vi "XNET String To IO Name (LIN Schedule Entry).vi"(3 "string":string) -> (0 "XNET LIN schedule entry":refnum<k21>)   [LabVIEW 2018]
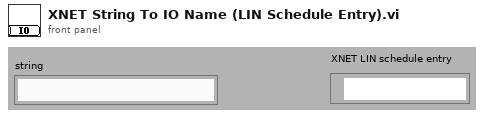
[diagram p1: front panel]
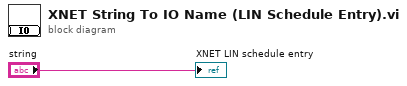
[diagram p0: block diagram]
diagram:
  "XNET LIN schedule entry" <- "string"
